vi "oa_Compute FFT Spectrum (1 Channel).vi"(7 "spectrum settings":cluster{"window type":u32, "block size":i32}={"window type"=1, "block size"=200} {"block size" min=2; "window type" items=["None"=0, "Hanning"=1, "Hamming"=2, "Blackman-Harris"=3, "Exact Blackman"=4, "Blackman"=5, "Flat Top"=6, "4 Term B-Harris"=7, "7 Term B-Harris"=8, "Low Sidelobe"=9, "Gaussian"=62]}, 10 "dr":dbl=1.0 format="%.2p", 11 "Y":dbl[][](array[numeric]) format="%.2f") -> (1 "df":dbl=1.0 format="%.2p", 3 "one-sided FFT spectrum":cdb[][](array[numeric]) format="%.2f")   [LabVIEW 2017, in "SoundVib_Resampling.lvlib"]
uses:
  <vilib>/addons/Sound and Vibration/Order Analysis/Resample Order Tracking/SoundVib_Resampling.lvlib
  <vilib>/Analysis/2dsp.llb/Real FFT.vi
  <vilib>/Analysis/NI_AALPro.lvlib
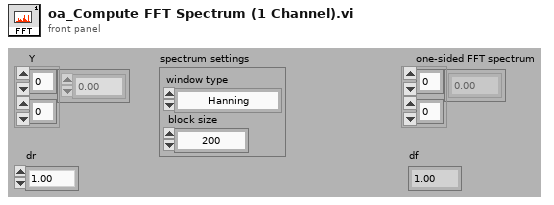
[diagram p1: front panel]
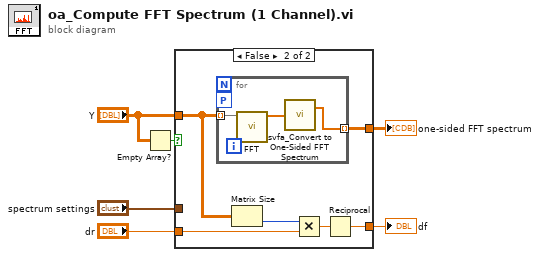
[diagram p0: block diagram]
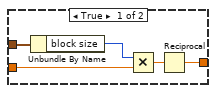
[diagram p2: hidden frame]
diagram:
  n1 = Empty Array?(array="Y") -> (empty?=w3:bool)
  n2 = case shown="False" w3 {
    tunnel: "Y" -> [_ w13]
    tunnel: [_ w16] -> w6
    tunnel: "dr" -> [w10 w15]
    tunnel: "spectrum settings" -> [w9 _]
    tunnel: [w7 w14] -> w1
    frame True {
      n3 = Unbundle By Name(w9) -> ("block size"=w8:i32)
      n4 = Multiply(x=w8, y=w10) -> (x*y=w11:dbl)
      n5 = Reciprocal(x=w11) -> (1/x=w7:dbl)
    }
    frame False {
      n6 = for {
        tunnel: w13 -> [w20] mode=indexing
        tunnel: [w18] -> w16 mode=indexing
        workers-P: _ -> [_]
        n7 = call-poly <vilib>:"FFT.vi"("X"=w20) -> ("FFT {X}"=w19:cdb[])  [unwired: 9 in, 1 out]
        n8 = call <vilib>:"svfa_Convert to One-Sided FFT Spectrum.vi"("two-sided FFT spectrum"=w19) -> ("one-sided FFT spectrum"=w18:cdb[])  [unwired: 1 out]
      }
      n9 = Matrix Size(0:w13) -> (2:w12:i32)  [unwired: 1 out]
      n10 = Multiply(x=w12, y=w15) -> (x*y=w17:dbl)
      n11 = Reciprocal(x=w17) -> (1/x=w14:dbl)
    }
  }
  "one-sided FFT spectrum" <- w6
  "df" <- w1
